vi "Read_Bypass.vi"(8 "error in (no error)":errorcluster, 11 "AccelNET.lvlib:TCP.lvclass":refnum<class "TCP.lvclass">) -> (0 "Error Out":errorcluster, 2 "Pelletron Bypass":T1)   [LabVIEW 2012, in "AccelNET.lvlib" / "TCP.lvclass"]
uses:
  TCP.lvclass
  Bypass_Indicator.ctl
  Read_Selector.ctl
  Useful_Controls.lvlib
  Useful_SubVIs.lvlib
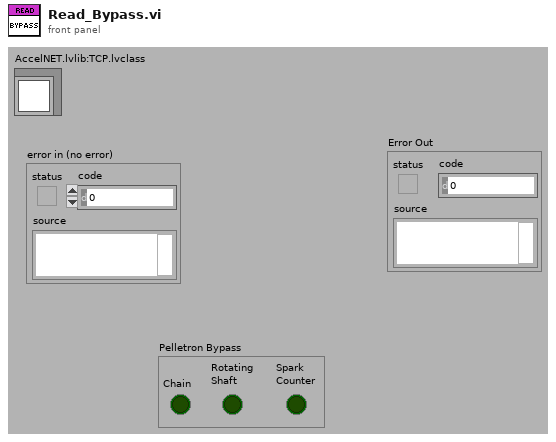
[diagram p1: front panel]
types:
  T1 = typedef "AccelNET.lvlib/Useful_Controls.lvlib/Bypass_Indicator.ctl" = cluster{"Chain":bool, "Rotating\nShaft":bool, "Spark\nCounter":bool}
  T2 = typedef "AccelNET.lvlib/Useful_Controls.lvlib/Read_Selector.ctl" = u16
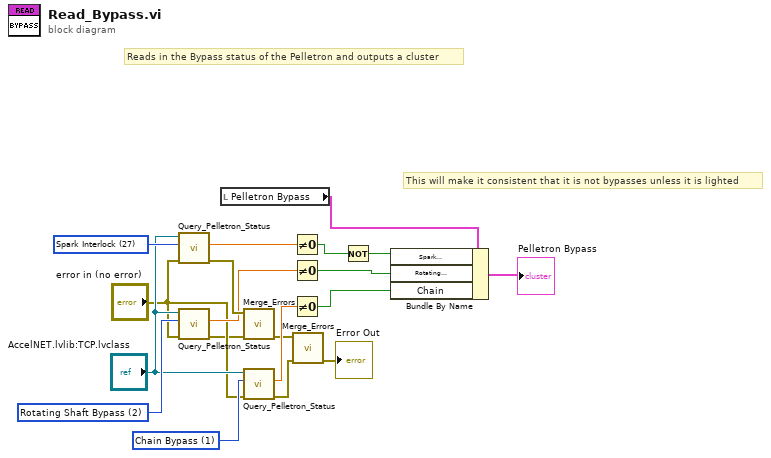
[diagram p0: block diagram]
diagram:
  w12 = T2 1 items=["Facility Key", "Chain Bypass", "Rotating Shaft Bypass", "Facility Interlock", "Pressure Interlock", "Temperature Interlock", "Water Flow Interlock", "Blower Status", "High Voltage", "+ High Voltage PS Readout", "- High Voltage PS Readout", "High Voltage PS Setting", "Ion Gauge", "Ion Filament", "Control Reference Voltage", "Control Mode", "Power Supply", "Chain Current", "Column Current", "Lost Current", "High Voltage Power Supply", "Rotating Shaft", "Chain", "Beamline GV", "Radiation", "Spark Count", "Spark Limit", "Spark Interlock"] ("Read Selector")
  w14 = T2 2 items=["Facility Key", "Chain Bypass", "Rotating Shaft Bypass", "Facility Interlock", "Pressure Interlock", "Temperature Interlock", "Water Flow Interlock", "Blower Status", "High Voltage", "+ High Voltage PS Readout", "- High Voltage PS Readout", "High Voltage PS Setting", "Ion Gauge", "Ion Filament", "Control Reference Voltage", "Control Mode", "Power Supply", "Chain Current", "Column Current", "Lost Current", "High Voltage Power Supply", "Rotating Shaft", "Chain", "Beamline GV", "Radiation", "Spark Count", "Spark Limit", "Spark Interlock"] ("Read Selector")
  w17 = T2 27 items=["Facility Key", "Chain Bypass", "Rotating Shaft Bypass", "Facility Interlock", "Pressure Interlock", "Temperature Interlock", "Water Flow Interlock", "Blower Status", "High Voltage", "+ High Voltage PS Readout", "- High Voltage PS Readout", "High Voltage PS Setting", "Ion Gauge", "Ion Filament", "Control Reference Voltage", "Control Mode", "Power Supply", "Chain Current", "Column Current", "Lost Current", "High Voltage Power Supply", "Rotating Shaft", "Chain", "Beamline GV", "Radiation", "Spark Count", "Spark Limit", "Spark Interlock"] ("Read Selector")
  # "This will make it consistent that it is not bypasses unless it is lighted"
  # "Reads in the Bypass status of the Pelletron and outputs a cluster"
  n1 = call "Query_Pelletron_Status.vi"("error in (no error)"="error in (no error)", "Read Selector"=w17, "AccelNET.lvlib:TCP.lvclass"="AccelNET.lvlib:TCP.lvclass") -> ("error out"=w16:errorcluster, "Data Out"=w18:dbl)  [unwired: 7 in]
  n2 = call "Query_Pelletron_Status.vi"("error in (no error)"="error in (no error)", "Read Selector"=w14, "AccelNET.lvlib:TCP.lvclass"="AccelNET.lvlib:TCP.lvclass") -> ("error out"=w7:errorcluster, "Data Out"=w15:dbl)  [unwired: 7 in]
  n3 = local read "Pelletron Bypass"() -> (w19:T1)
  n4 = call "Merge_Errors.vi"("Error 2"=w7, "Error 1"=w16) -> ("Error Out"=w5:errorcluster)  [unwired: 9 in]
  n5 = call "Query_Pelletron_Status.vi"("error in (no error)"="error in (no error)", "Read Selector"=w12, "AccelNET.lvlib:TCP.lvclass"="AccelNET.lvlib:TCP.lvclass") -> ("error out"=w6:errorcluster, "Data Out"=w13:dbl)  [unwired: 7 in]
  n6 = Not Equal To 0?(x=w18) -> (x != 0?=w2:bool)
  n7 = Not Equal To 0?(x=w15) -> (x != 0?=w8:bool)
  n8 = Not Equal To 0?(x=w13) -> (x != 0?=w9:bool)
  n9 = call "Merge_Errors.vi"("Error 2"=w6, "Error 1"=w5) -> ("Error Out"=→"Error Out":errorcluster)  [unwired: 9 in]
  n10 = Not(x=w2) -> (.not. x?=w1:bool)
  n11 = Bundle By Name(cluster=w19, "Spark\nCounter"=w1, "Rotating\nShaft"=w8, "Chain"=w9) -> (→"Pelletron Bypass":T1)
